vi "Test App Processes Receive all calls.vi"(8 "error in (no error)":errorcluster, 11 "Rig Test In":refnum<class "Application Test.lvclass">) -> (0 "error out":errorcluster, 3 "Rig Test Out":refnum<class "Application Test.lvclass">)   [LabVIEW 2020, in "Application Test.lvclass"]
uses:
  Application Test.lvclass
  C:/Program Files (x86)/National Instruments/LabVIEW 2020/vi.lib/Asteme/LUnit/Test Case.lvclass
  Mock Process/Mock Process.lvclass
  C:/Users/anton/Documents/GitHub/Triarc-Framework/source/Framework/Process/Process.lvclass
  Framework/Process/Process.lvclass/Process.ctl
  Framework/Application/Application.lvclass/Application.ctl
  <vilib>/Asteme/LUnit/Test Case.lvclass/Test Case.ctl
  <vilib>/Asteme/LUnit/LUnit Assertion Result.lvclass/LUnit Assertion Result.ctl
  Framework/Application/Private/Add Process to Map.vi
  Framework/Application/Private/Start Idle Processes if Running.vi
  Framework/Process/Protected/Messaging/Enqueue Message.vi
  Framework/Process/Public/Lifecycle/Get Lifecycle State.vi
  Framework/Process/Protected/SubVIs/Set Context.vi
  Framework/Process/Private/SubVIs/Wait for finish.vi
  Framework/Process/Private/SubVIs/Set Lifecycle State.vi
  <vilib>/Asteme/LUnit/Palette/Fail.vi
  <vilib>/Asteme/LUnit/Palette/Pass.vi
  <vilib>/Asteme/LUnit/Set Assertion Type.vi
  <vilib>/Utility/error.llb/Clear Errors.vi
  Framework/Process/Public/Lifecycle/Leave Process Loop.vi
  <vilib>/Asteme/LUnit/Add test result.vi
  <vilib>/Asteme/LUnit/LUnit Write Passed.vi
  <vilib>/Asteme/LUnit/LUnit Get Test Case.vi
  <vilib>/Asteme/LUnit/Assertion Result/LUnit Get Test Name.vi
  <vilib>/Asteme/LUnit/LUnit Write Message.vi
  <vilib>/Asteme/LUnit/LUnit Write Description.vi
  <vilib>/Asteme/LUnit/LUnit Write Assertion Type.vi
  <vilib>/Asteme/LUnit/Read Test Case Name.vi
  Framework/Application/Application.lvclass
  <vilib>/Utility/error.llb/Error Cluster From Error Code.vi
  Framework/Application/Private/Update Context for Owned Processes.vi
  <vilib>/Asteme/LUnit/LUnit Assertion Result.lvclass
  Framework/Process/Process.lvclass
  <vilib>/Asteme/LUnit/Test Case.lvclass
panel:
  out "Messages":string[](array[string])
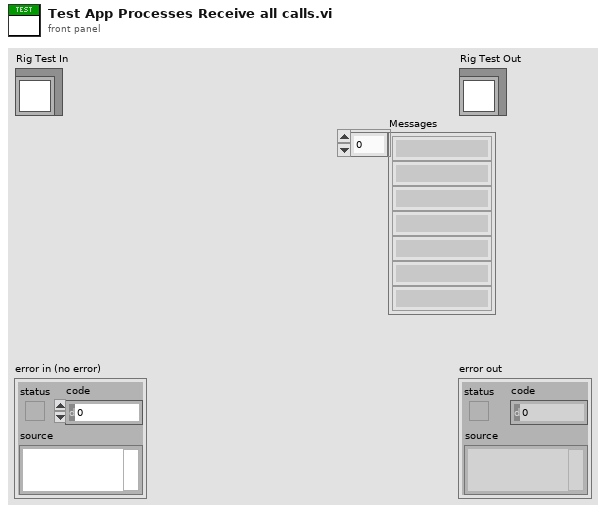
[diagram p1: front panel]
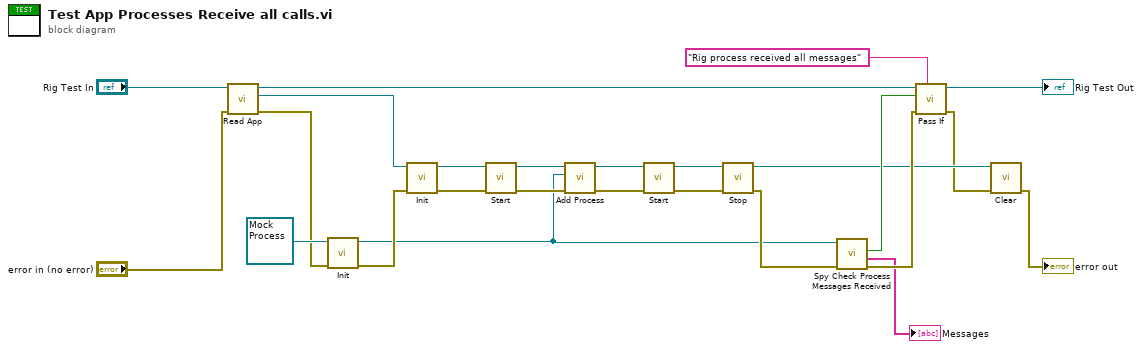
[diagram p0: block diagram]
diagram:
  n1 = call "Read App.vi"("error in (no error)"="error in (no error)", "Application Test In"="Rig Test In") -> ("error out"=w8:errorcluster, "App out"=w9:refnum<class "Application.lvclass">, "Application Test Out"=w24:refnum<class "Application Test.lvclass">)  [unwired: 7 in]
  n2 = call-dynamic "Init.vi"("error in (no error)"=w8, "Mock Process In"=refnum<class "Mock Process.lvclass"> refnum ("Mock Classes.lvlib:Mock Process.lvclass")) -> ("error out"=w14:errorcluster, "Mock Process Out"=w10:refnum<class "Mock Process.lvclass">)  [unwired: 8 in]
  n3 = call-dynamic "Init.vi"("error in (no error)"=w14, "Process In"=w9) -> ("error out"=w21:errorcluster, "Process Out"=w22:refnum<class "Application.lvclass">)  [unwired: 8 in]
  n4 = call "Start.vi"("error in (no error)"=w21, "Process In"=w22) -> ("error out"=w20:errorcluster, "Process Out"=w16:refnum<class "Application.lvclass">)  [unwired: 8 in]
  n5 = call "Add Process.vi"("error in (no error)"=w20, "Process"=w10, "Rig In"=w16) -> ("error out"=w7:errorcluster, "Rig Out"=w6:refnum<class "Application.lvclass">)  [unwired: 7 in]
  n6 = call "Start.vi"("error in (no error)"=w7, "Process In"=w6) -> ("error out"=w18:errorcluster, "Process Out"=w19:refnum<class "Application.lvclass">)  [unwired: 8 in]
  n7 = call "Stop.vi"("error in (no error)"=w18, "Process In"=w19) -> ("error out"=w17:errorcluster, "Process Out"=w3:refnum<class "Application.lvclass">)  [unwired: 7 in, 1 out]
  n8 = call "Spy Check Process Messages Received.vi"("error in (no error)"=w17, "Mock Process In"=w10) -> ("error out"=w5:errorcluster, "Messages"=→"Messages":string[], "Messages received?"=w12:bool)  [unwired: 6 in, 1 out]
  n9 = call <vilib>:"Pass If.vi"("Description"="Rig process received all messages", "error in (no error)"=w5, "Pass?"=w12, "Test Case In"=w24) -> ("error out"=w2:errorcluster, "Test Case Out"=→"Rig Test Out":refnum<class "Application Test.lvclass">)  [unwired: 6 in]
  n10 = call-dynamic "Clear.vi"("error in (no error)"=w2, "Application In"=w3) -> ("error out"=→"error out":errorcluster)  [unwired: 9 in]
